vi "XY to 2D.vi"(8 "error in (no error)":errorcluster, 9 "Fake Point":dbl, 10 "Interpolate [T]":bool=TRUE, 11 "XY-data":cluster{"X-array":dbl[], "Y-array":dbl[]}[](array[cluster]) {"Y-array" format="%.2p"; "X-array" format="%.2p"}) -> (0 "error out":errorcluster, 1 "Interpolated XY-data out":cluster{"X-array":dbl[], "Y-array":dbl[]}[](array[cluster]), 2 "X Array":dbl[](array[numeric]), 3 "2D Y Array":dbl[][](array[numeric]))   [LabVIEW 2019, in "xy_utilities.lvlib"]
doc: "Interpolate Array of <b>XY-Data</b> to <b>2D Y Array</b> and <b>X Array</b>"
uses:
  xy_utilities.lvlib
  <vilib>/Analysis/NI_AALBase.lvlib
  subVIs/Get X and Y (single).vi
  Typedefs/Interpolation Configuration--cluster.ctl
  subVIs/Interpolate (multiple).vi
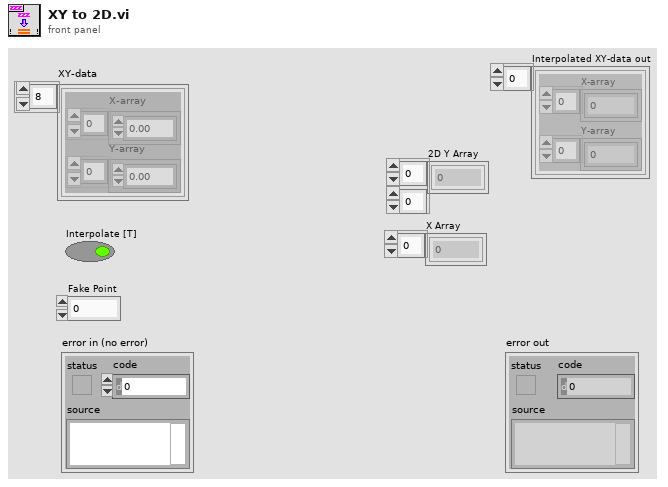
[diagram p1: front panel]
types:
  T1 = typedef "xy_utilities.lvlib/Interpolation Configuration--cluster.ctl" = cluster{"X Low":dbl, "X High":dbl, "X Step":dbl, "Fake Point":dbl}
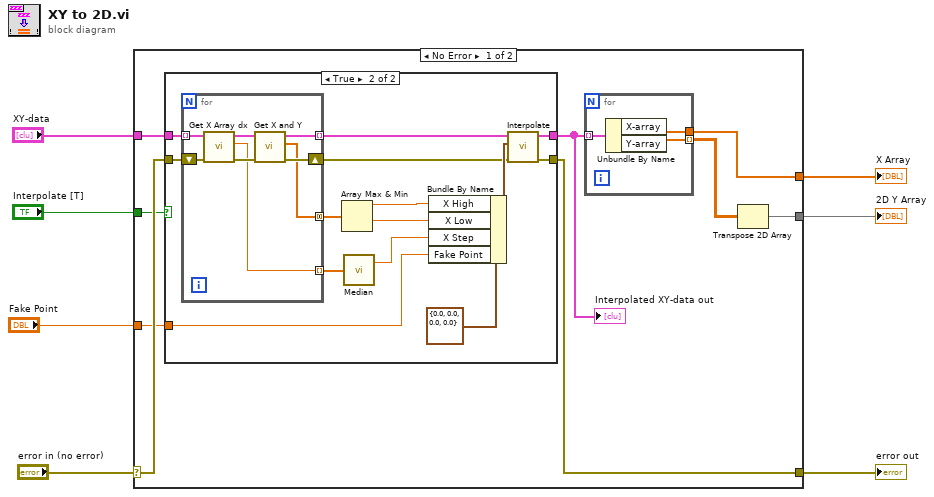
[diagram p0: block diagram]
diagram:
  n1 = case shown="No Error" "error in (no error)" {
    selector: "error in (no error)" -> [w13 w44]
    tunnel: [w16 w44] -> w6
    tunnel: "XY-data" -> [w14 _]
    tunnel: [w11 _] -> w4
    tunnel: [w15 _] -> w3
    tunnel: "Interpolate [T]" -> [w12 _]
    tunnel: "Fake Point" -> [w8 _]
    frame No Error {
      n2 = case shown="True" w12 {
        tunnel: [w18 w29] -> w9
        tunnel: [w17 w27] -> w16
        tunnel: w14 -> [w18 w25]
        tunnel: w13 -> [w17 w23]
        tunnel: w8 -> [_ w20]
        frame False {
        }
        frame True {
          n3 = for {
            tunnel: w25 -> [w40] mode=indexing
            tunnel: [w33] -> w28 mode=concatenating
            tunnel: [w37] -> w26 mode=indexing
            tunnel: [w36] -> w24 mode=indexing
            shift-right: [w35] -> w22
            shift-left: w23 -> [w34]
            n4 = call "Get X Array dx.vi"("error in (no error)"=w34, "XY-data"=w40) -> ("error out"=w38:errorcluster, "dX"=w37:dbl, "XY-data out"=w39:cluster{"X-array":dbl[], "Y-array":dbl[]})  [unwired: 6 in, 1 out]
            n5 = call-poly "Get X and Y.vi"("error in (no error)"=w38, "XY-data"=w39) -> ("error out"=w35:errorcluster, "X-array"=w33:dbl[], "XY-data out"=w36:cluster{"X-array":dbl[], "Y-array":dbl[]})  [unwired: 6 in, 1 out]
          }
          n6 = Array Max & Min(array=w28) -> (max value=w31:dbl, min value=w32:dbl)  [unwired: 2 out]
          n7 = call <vilib>:"Median.vi"("X"=w26) -> ("median"=w19:dbl)  [unwired: 1 out]
          n8 = Bundle By Name(cluster=T1 {"X Low"=0.0, "X High"=0.0, "X Step"=0.0, "Fake Point"=0.0} ("Configure"), "X High"=w31, "X Low"=w32, "X Step"=w19, "Fake Point"=w20) -> (w30:T1)
          n9 = call-poly "Interpolate.vi"("error in (no error)"=w22, "Configure"=w30, "XY-data"=w24) -> ("error out"=w27:errorcluster, "Interpolated XY-data out"=w29:cluster{"X-array":dbl[], "Y-array":dbl[]}[])  [unwired: 7 in]
        }
      }
      "Interpolated XY-data out" <- w9
      n10 = for {
        tunnel: w9 -> [w43] mode=indexing
        tunnel: [w42] -> w10 mode=indexing
        tunnel: [w41] -> w15
        n11 = Unbundle By Name(w43) -> ("X-array"=w41:dbl[], "Y-array"=w42:dbl[])
      }
      n12 = Transpose 2D Array(2D array=w10) -> (transposed array=w11:dbl[][])
    }
    frame Error {
    }
  }
  "error out" <- w6
  "2D Y Array" <- w4
  "X Array" <- w3
